vi "数字识别.vi"(2 "Exit Event":refnum<user-event>) -> ()   [LabVIEW 2018]
uses:
  <vilib>/userdefined/High Color/IMAQdx.ctl
  <vilib>/vision/Image Controls.llb/IMAQ Image.ctl
  <vilib>/vision/driver/IMAQdx.llb/IMAQdx Acquisition Mode.ctl
  <vilib>/vision/NI_Vision_Development_Module.lvlib
  <vilib>/vision/driver/NI_Vision_Acquisition_Software.lvlib
panel:
  in  "Session In":T1
  in  "开始":bool
  in  "静态 / 实时":bool
  in  "stop":bool
  out "识别的文字":string
  out "Image Out":T2(plugin-control)
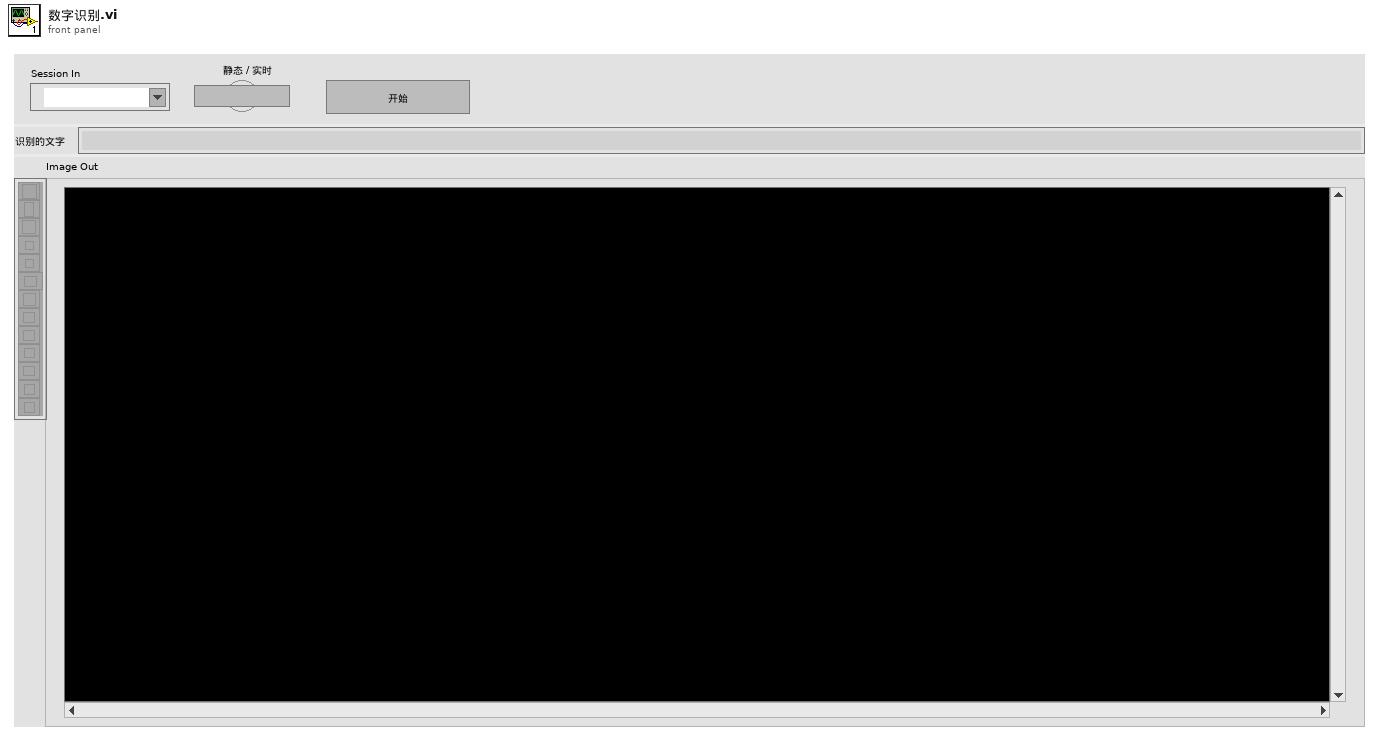
[diagram p1: front panel]
types:
  T1 = typedef "IMAQdx.ctl" = refnum<k21>
  T2 = typedef "IMAQ Image.ctl" = refnum<image>
  T3 = enum8{"Enabled", "Disabled", "Disabled and Grayed Out"}
  T4 = cluster{"Threshold Mode":i32, "Fixed Threshold Range":cluster{"Lower value":sgl, "Upper value":sgl}, "Advanced Threshold Data":cluster{"Number of Blocks":i32, "Pixel Value Range":cluster{"Lower value":i32, "Upper value":i32}, "Optimize For Speed":bool, "Perform Bi-modal Calculation":bool}, "Character Color":i32, "Reject Border":bool, "Number Of Erosions":i32, "Size & Spacing":cluster{"AutoSplit":bool, "Min Bounding Rect Width":i32, "Max Bounding Rect Width":i32, "Min Bounding Rect Height":i32, "Max Bounding Rect Height":i32, "Min Character Size":i32, "Max Character Size":i32, "Min Char Spacing":i32, "Max Horiz Element Spacing":i32, "Max Vert Element Spacing":i32}, "Read Options":cluster{"Read Strategy":i32, "Read Resolution":i32, "Scale Dependant":bool, "Aspect Ratio":i32, "Acceptance Level":i32, "Substitution Character":string}, "Valid Characters":cluster{"Pre-defined characters":i32, "User-defined characters":string}[], "Use Text Pattern":bool, "Orientation":u32}
  T5 = typedef "NI_Vision_Acquisition_Software.lvlib/IMAQdx Acquisition Mode.ctl" = enum32{"One Shot", "Continuous"}
  T6 = typedef "Image Type" = u32
  T7 = typedef "IMAQ OCR Session.ctl" = refnum<k1>
  T8 = cluster{"Global Rectangle":i32[], "Contours":cluster{"Contour Type":u32, "ROI Type":u32, "Points":i32[]}[]}
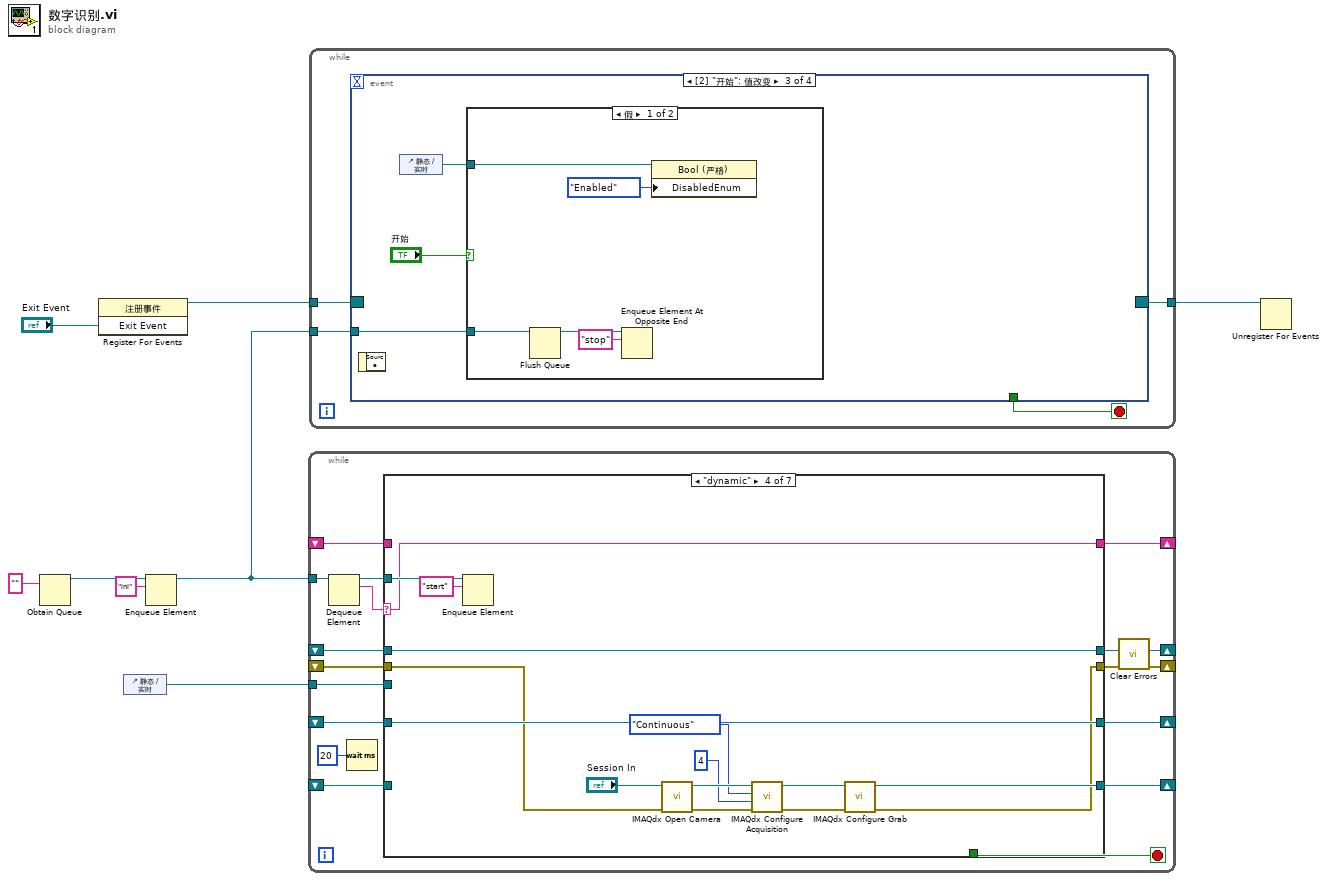
[diagram p0: block diagram]
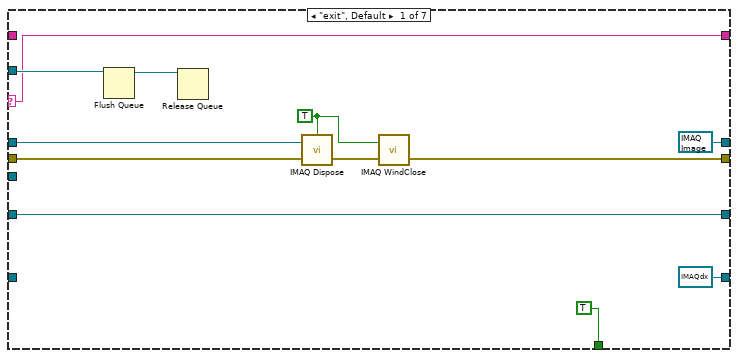
[diagram p2: hidden frame]
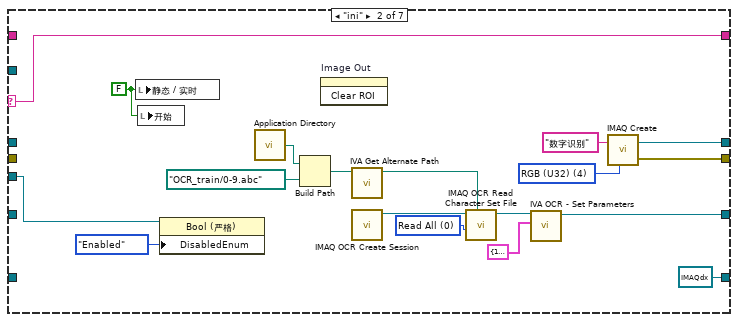
[diagram p3: hidden frame]
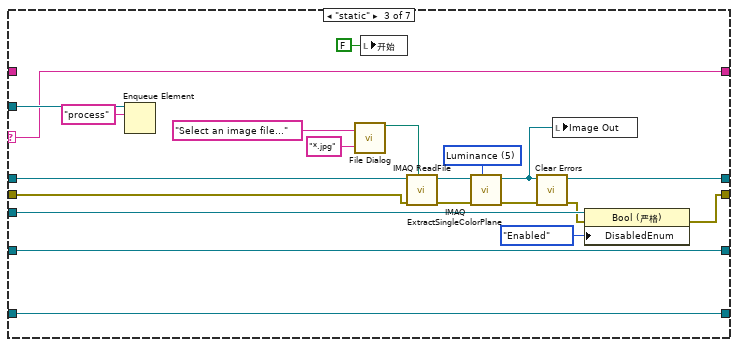
[diagram p4: hidden frame]
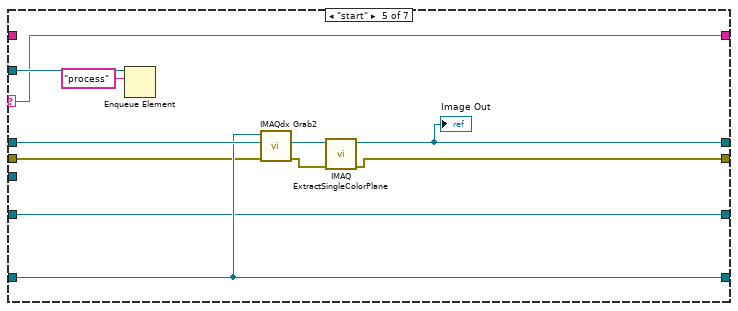
[diagram p5: hidden frame]
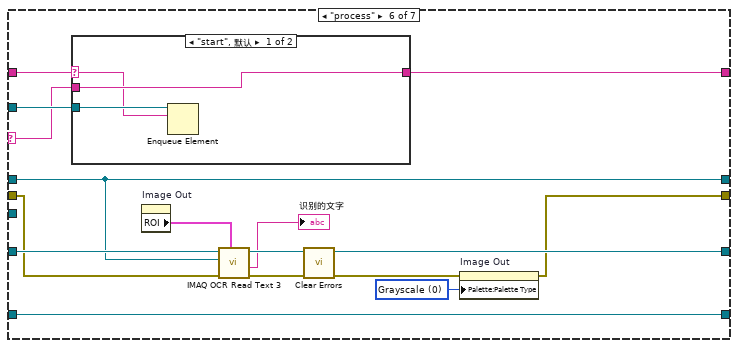
[diagram p6: hidden frame]
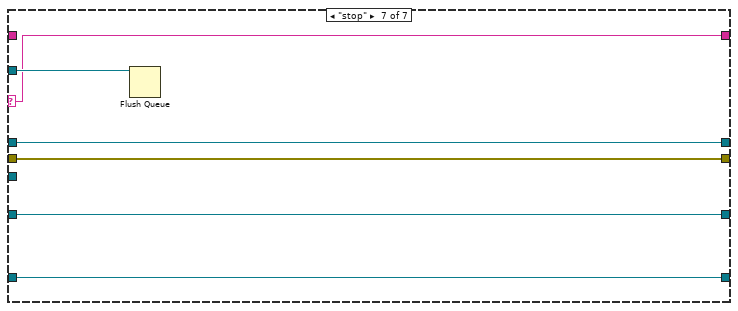
[diagram p8: hidden frame]
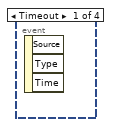
[diagram p9: hidden frame]
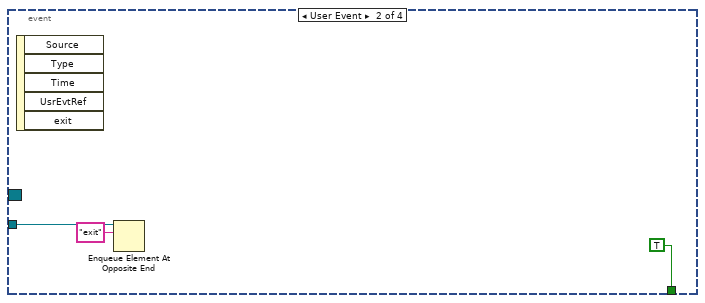
[diagram p10: hidden frame]
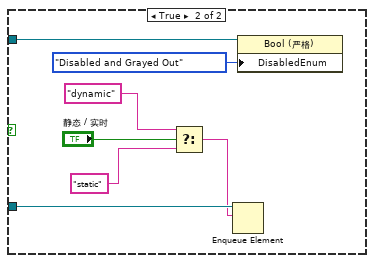
[diagram p11: hidden frame]
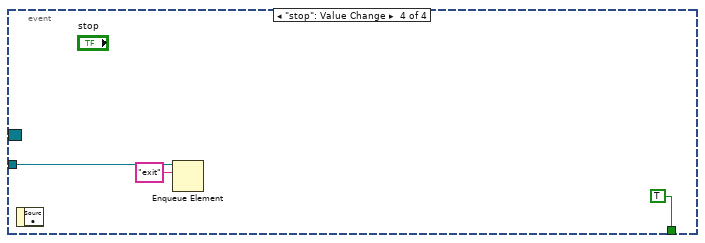
[diagram p12: hidden frame]
diagram:
  n1 = Obtain Queue(element data type="") -> (queue out=w5:refnum<queue>)  [unwired: 4 in, 2 out]
  n2 = register-events("Exit Event") -> (reference out=w2:refnum<event-registration>)  [unwired: 2 in, 1 out]
  n3 = control-ref of="静态 / 实时"() -> (w1:refnum<vi>)
  n4 = Enqueue Element(queue=w5, element="ini") -> (queue out=w3:refnum<queue>)  [unwired: 2 in, 2 out]
  n5 = while {
    tunnel: w3 -> [w25]
    shift-right: [w21] -> _
    shift-left: _ -> [w20]
    shift-right: [w19] -> _
    shift-left: _ -> [w18]
    shift-right: [w17] -> _
    shift-left: _ -> [w16]
    shift-right: [w15] -> _
    shift-left: _ -> [w14]
    tunnel: w1 -> [w13]
    shift-right: [w10] -> _
    shift-left: _ -> [w11]
    stop <- w22 stop-if-true
    n6 = Dequeue Element(queue=w25) -> (queue out=w23:refnum<queue>, element=w24:string)  [unwired: 2 in, 2 out]
    n7 = Wait (ms)(milliseconds to wait=u32 20 ("等待时间（毫秒）")) -> ()  [unwired: 1 out]
    n8 = case shown="\"dynamic\"" w24 {
      selector: w24 -> [w28 w45 w65 w87 w97 w108 w123]
      tunnel: w23 -> [w37 _ w68 w89 w98 w109 w126]
      tunnel: [TRUE _ _ _ _ _ _] -> w22
      tunnel: [T2 refnum ("New Image") w42 w69 w90 w94 w110 w125] -> w21
      tunnel: w20 -> [w32 _ w63 w90 w100 w110 w125]
      tunnel: [T1 refnum ("Session Out") T1 refnum ("Session Out") w75 w79 w99 w116 w124] -> w19
      tunnel: w18 -> [_ _ w75 _ w99 w116 w124]
      tunnel: [w29 w46 w66 w86 w96 w111 w122] -> w17
      tunnel: w16 -> [w29 _ w66 w86 w96 w112 w122]
      tunnel: [w28 w45 w65 w87 w97 w107 w123] -> w15
      tunnel: w14 -> [_ _ _ _ _ w106 _]
      tunnel: w13 -> [_ w40 w62 _ _ _ _]
      tunnel: [w27 w38 w59 w77 w91 w102 w121] -> w12
      tunnel: w11 -> [w26 _ w56 w76 w93 w104 w121]
      frame "exit", Default {
        w33 = TRUE ("All Images? (No)")
        n9 = Flush Queue(queue=w37) -> (queue out=w36:refnum<queue>)  [unwired: 1 in, 2 out]
        n10 = Release Queue(queue=w36) -> ()  [unwired: 2 in, 3 out]
        n11 = call "IMAQ Dispose"("All Images? (No)"=w33, "Image"=w32, "error in (no error)"=w26) -> ("error out"=w34:errorcluster)  [unwired: 3 in]
        n12 = call "IMAQ WindClose"("Close All Windows (False)"=w33, "error in (no error)"=w34) -> ("error out"=w27:errorcluster)  [unwired: 4 in]
      }
      frame "ini" {
        w41 = FALSE ("静态 / 实时")
        w44 = T6 4 items=["Grayscale (U8)", "Grayscale (I16)", "Grayscale (SGL)", "Complex (CSG)", "RGB (U32)", "HSL (U32)", "RGB (U64)", "Grayscale (U16)"] ("Image Type")
        w50 = 0 items=["Read All", "Read Character Set Only", "Read Properties Only"] ("Read Options")
        n13 = local write "静态 / 实时"(w41) -> ()
        n14 = local write "开始"(w41) -> ()
        n15 = property class="Bool (严格)"(reference=w40, "DisabledEnum"=T3."Enabled" ("Disabled")) -> ()  [unwired: 1 in, 2 out]
        n16 = call <vilib>:"Application Directory.vi"() -> ("Application Directory"=w49:path)
        n17 = Build Path(base path=w49, name or relative path=path "OCR_train/0-9.abc") -> (appended path=w47:path)
        n18 = invoke on="Image Out" class="ImageControl" method="Clear ROI"() -> ()  [unwired: 3 in, 3 out]
        n19 = call <vilib>:"IVA Get Alternate Path.vi"("Path In"=w47) -> ("Path Out"=w54:path)  [unwired: 10 out]
        n20 = call "IMAQ OCR Create Session"() -> ("IMAQ OCR Session"=w52:T7)  [unwired: 1 in, 10 out]
        n21 = call "IMAQ OCR Read Character Set File"("File Path"=w54, "Read Options"=w50, "IMAQ OCR Session"=w52) -> ("IMAQ OCR Session (dup)"=w53:T7)  [unwired: 2 in, 6 out]
        n22 = call <vilib>:"IVA OCR - Set Parameters.vi"("Parameters"=T4 {"Threshold Mode"=1, "Fixed Threshold Range"={"Lower value"=1.0, "Upper value"=255.0}, "Advanced Threshold Data"={"Number of Blocks"=4, "Pixel Value Range"={"Lower value"=0, "Upper value"=255}, "Optimize For Speed"=FALSE, "Perform Bi-modal Calculation"=FALSE}, "Character Color"=0, "Reject Border"=FALSE, "Number Of Erosions"=0, "Size & Spacing"={"AutoSplit"=FALSE, "Min Bounding Rect Width"=1, "Max Bounding Rect Width"=65536, "Min Bounding Rect Height"=1, "Max Bounding Rect Height"=65536, "Min Character Size"=20, "Max Character Size"=65536, "Min Char Spacing"=1, "Max Horiz Element Spacing"=1, "Max Vert Element Spacing"=0}, "Read Options"={"Read Strategy"=1, "Read Resolution"=2, "Scale Dependant"=FALSE, "Aspect Ratio"=400, "Acceptance Level"=700, "Substitution Character"="?"}, "Valid Characters"=[], "Use Text Pattern"=FALSE, "Orientation"=0} ("Parameters (OCR/OCV 1)"), "IMAQ OCR Session"=w53) -> ("IMAQ OCR Session Out"=w46:T7)  [unwired: 1 in, 8 out]
        n23 = call "IMAQ Create"("Image Name"="数字识别", "Image Type"=w44) -> ("New Image"=w42:T2, "error out"=w38:errorcluster)  [unwired: 2 in, 1 out]
      }
      frame "static" {
        w72 = 5 items=["Red", "Green", "Blue", "Hue", "Saturation", "Luminance", "Value", "Intensity"] ("Color Plane")
        n24 = Enqueue Element(queue=w68, element="process") -> ()  [unwired: 2 in, 3 out]
        n25 = call "File Dialog"("prompt"="Select an image file...", "pattern (all files)"="*.jpg") -> ("selected path"=w74:path)  [unwired: 5 in, 8 out]
        n26 = local write "开始"(FALSE ("开始")) -> ()
        n27 = call "IMAQ ReadFile"("File Path"=w74, "error in (no error)"=w56, "Image"=w63) -> ("error out"=w57:errorcluster, "Image Out"=w73:T2)  [unwired: 2 in, 5 out]
        n28 = call "IMAQ ExtractSingleColorPlane"("Color Plane"=w72, "error in (no error)"=w57, "Image Src"=w73) -> ("error out"=w60:errorcluster, "Image Dst Out"=w69:T2)  [unwired: 1 in, 6 out]
        n29 = call <vilib>:"Clear Errors.vi"("error in (no error)"=w60) -> ("error out"=w58:errorcluster)  [unwired: 5 in, 1 out]
        n30 = local write "Image Out"(w69) -> ()
        n31 = property class="Bool (严格)"(reference=w62, error in=w58, "DisabledEnum"=T3."Enabled" ("Disabled")) -> (error out=w59:errorcluster)  [unwired: 1 out]
      }
      frame "dynamic" {
        n32 = Enqueue Element(queue=w89, element="start") -> ()  [unwired: 2 in, 3 out]
        n33 = call <vilib>:"IMAQdx Open Camera.vi"("error in"=w76, "Session In"="Session In") -> ("error out"=w80:errorcluster, "Session Out"=w85:T1)  [unwired: 8 in]
        n34 = call <vilib>:"IMAQdx Configure Acquisition.vi"("error in"=w80, "Number of Buffers"=u32 4, "Continuous?"=IMAQdx_Acquisition_Mode."Continuous", "Session In"=w85) -> ("error out"=w81:errorcluster, "Session Out"=w82:T1)  [unwired: 6 in]
        n35 = call <vilib>:"IMAQdx Configure Grab.vi"("error in"=w81, "Session In"=w82) -> ("error out"=w77:errorcluster, "Session Out"=w79:T1)  [unwired: 8 in]
      }
      frame "start" {
        n36 = Enqueue Element(queue=w98, element="process") -> ()  [unwired: 2 in, 3 out]
        n37 = call <vilib>:"IMAQdx Grab2.vi"("error in"=w93, "Image In"=w100, "Session In"=w99) -> ("error out"=w92:errorcluster, "Image Out"=w101:T2)  [unwired: 5 in, 2 out]
        n38 = call "IMAQ ExtractSingleColorPlane"("error in (no error)"=w92, "Image Src"=w101) -> ("error out"=w91:errorcluster, "Image Dst Out"=w94:T2)  [unwired: 8 in]
        "Image Out" <- w94
      }
      frame "process" {
        w113 = u32 0 items=["Grayscale", "Binary", "Gradient", "Rainbow", "Temperature", "User Defined"] ("Palette")
        n39 = case shown="\"start\", 默认" w106 {
          selector: w106 -> [w117 _]
          tunnel: w109 -> [w119 _]
          tunnel: w108 -> [w118 w120]
          tunnel: [w118 w120] -> w107
          frame "start", Default {
            n40 = Enqueue Element(queue=w119, element=w117) -> ()  [unwired: 2 in, 3 out]
          }
          frame "static" {
          }
        }
        n41 = property on="Image Out" class="ImageControl"() -> ("ROI"=w115:T8)  [unwired: 2 in, 2 out]
        n42 = call "IMAQ OCR Read Text 3"("ROI Descriptor"=w115, "error in (no error)"=w104, "Image"=w110, "IMAQ OCR Session"=w112) -> ("error out"=w114:errorcluster, "Read String"=→"识别的文字":string, "IMAQ OCR Session (dup)"=w111:T7)  [unwired: 1 in, 4 out]
        n43 = call <vilib>:"Clear Errors.vi"("error in (no error)"=w114) -> ("error out"=w103:errorcluster)  [unwired: 5 in, 1 out]
        n44 = property on="Image Out" class="ImageControl"(error in=w103, "Palette:Palette Type"=w113) -> (error out=w102:errorcluster)  [unwired: 1 in, 1 out]
      }
      frame "stop" {
        n45 = Flush Queue(queue=w126) -> ()  [unwired: 1 in, 3 out]
      }
    }
    n46 = call <vilib>:"Clear Errors.vi"("error in (no error)"=w12) -> ("error out"=w10:errorcluster)  [unwired: 5 in, 1 out]
  }
  n47 = while {
    tunnel: w2 -> [w130]
    tunnel: [w129] -> w7
    tunnel: w3 -> [w127]
    stop <- w128 stop-if-true
    n48 = event shown="[2] \"开始\": 值改变" {
      selector: w130 -> [_ _ _ _]
      dyn-events: [_ _ _ _] -> w129
      timeout: _ -> [_ _ _ _]
      tunnel: [_ TRUE _ TRUE] -> w128
      tunnel: w127 -> [_ w132 w136 w150]
      event Timeout {
        n49 = event-data() -> ()  [unwired: 1 in, 3 out]
      }
      event User Event {
        n50 = event-data() -> ()  [unwired: 1 in, 5 out]
        n51 = Enqueue Element At Opposite End(queue=w132, element="exit") -> ()  [unwired: 2 in, 3 out]
      }
      event "开始": Value Change {
        n52 = event-data() -> ()  [unwired: 1 in, 1 out]
        n53 = control-ref of="静态 / 实时"() -> (w134:refnum<vi>)
        n54 = case shown="假" "开始" {
          tunnel: w136 -> [w141 w148]
          tunnel: w134 -> [w138 w143]
          frame False {
            n55 = Flush Queue(queue=w141) -> (queue out=w140:refnum<queue>)  [unwired: 1 in, 2 out]
            n56 = Enqueue Element At Opposite End(queue=w140, element="stop") -> ()  [unwired: 2 in, 3 out]
            n57 = property class="Bool (严格)"(reference=w138, "DisabledEnum"=T3."Enabled" ("Disabled")) -> ()  [unwired: 1 in, 2 out]
          }
          frame True {
            n58 = Select(t="dynamic" ("f"), s="静态 / 实时", f="static" ("element")) -> (s? t:f=w146:string)
            n59 = Enqueue Element(queue=w148, element=w146) -> ()  [unwired: 2 in, 3 out]
            n60 = property class="Bool (严格)"(reference=w143, "DisabledEnum"=T3."Disabled and Grayed Out" ("Disabled")) -> ()  [unwired: 1 in, 2 out]
          }
        }
      }
      event "stop": Value Change {
        n61 = event-data() -> ()  [unwired: 1 in, 1 out]
        n62 = Enqueue Element(queue=w150, element="exit") -> ()  [unwired: 2 in, 3 out]
      }
    }
  }
  n63 = Unregister For Events(event registration refnum=w7) -> ()  [unwired: 1 in, 1 out]
